vi "Power-on Setup.vi"(8 "error in (no error)":errorcluster, 10 "Power-on Setup (0: RST)":i32(ring) items=["RST", "Preset", "SAV0"], 11 "VISA resource name":refnum<visa-resource-name>) -> (0 "error out":errorcluster, 3 "VISA resource name out":refnum<visa-resource-name>)   [LabVIEW 2021, in "Keithley 2182.lvlib"]
doc: "Sets the power-on defaults."
uses:
  <instrlib>/Keithley 2182/Keithley 2182.lvlib
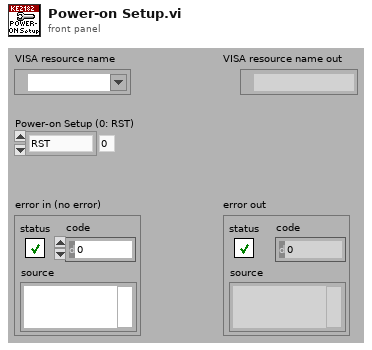
[diagram p1: front panel]
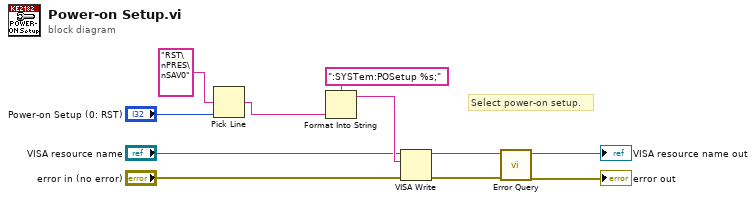
[diagram p0: block diagram]
diagram:
  # "Select power-on setup."
  n1 = Pick Line(multi-line string="RST\nPRES\nSAV0", line index="Power-on Setup (0: RST)") -> (output string=w2:string)  [unwired: 1 in]
  n2 = Format Into String(format string=":SYSTem:POSetup %s;", w2) -> (resulting string=w10:string)  [unwired: 2 in, 1 out]
  n3 = VISA Write(VISA resource name="VISA resource name", write buffer=w10, error in (no error)="error in (no error)") -> (VISA resource name out=w7:refnum<visa-resource-name>, error out=w6:errorcluster)  [unwired: 1 out]
  n4 = call <instrlib>:"Error Query.vi"("error in (no error)"=w6, "VISA resource name"=w7) -> ("error out"=→"error out":errorcluster, "VISA resource name out"=→"VISA resource name out":refnum<visa-resource-name>)  [unwired: 6 in, 2 out]
